vi "Activate Window.vi"(8 "error in (no error)":errorcluster, 11 "Hwnd":u32) -> (0 "error out":errorcluster)   [LabVIEW 2019, in "LV MDI.lvclass"]
uses:
  LV MDI.lvclass
  user32.dll
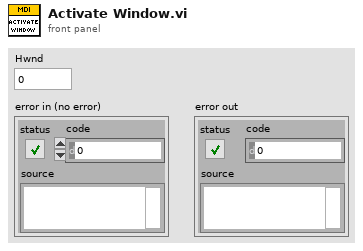
[diagram p1: front panel]
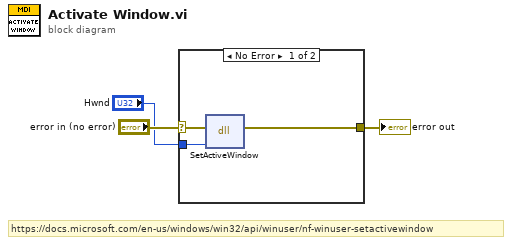
[diagram p0: block diagram]
diagram:
  # "https://docs.microsoft.com/en-us/windows/win32/api/winuser/nf-winuser-setactivewindow"
  n1 = case shown="No Error" "error in (no error)" {
    selector: "error in (no error)" -> [w6 w7]
    tunnel: [w5 w7] -> w2
    tunnel: "Hwnd" -> [w4 _]
    frame No Error {
      n2 = dll-call lib="user32.dll" fn="SetActiveWindow"(error in=w6, "hwnd"=w4) -> (error out=w5:errorcluster)  [unwired: 4 in, 1 out]
    }
    frame Error {
    }
  }
  "error out" <- w2
